vi "AB_UserComponentsPath.vi"(8 "error in (no error)":errorcluster) -> (0 "error out":errorcluster, 3 "path to User Components":path)   [LabVIEW 2020]
uses:
  <vilib>/registry/registry.llb/Registry View.ctl
  <vilib>/registry/registry.llb/Registry SAM.ctl
  <vilib>/registry/registry.llb/Registry RtKey.ctl
  <vilib>/registry/registry.llb/Read Registry Value Simple STR.vi
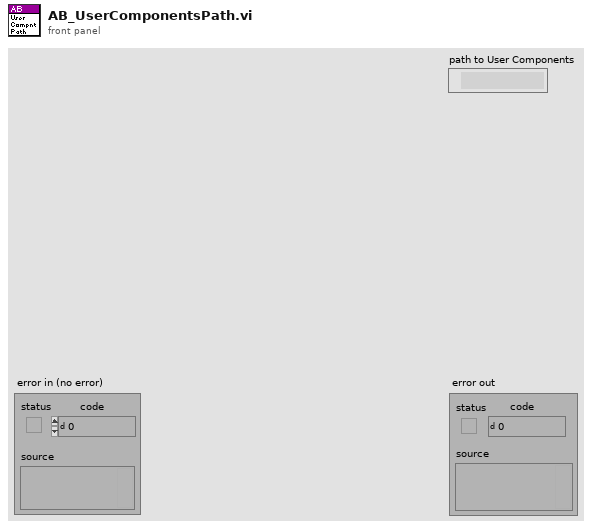
[diagram p1: front panel]
types:
  T1 = typedef "Registry RtKey.ctl" = enum32{"HKEY_CLASSES_ROOT", "HKEY_CURRENT_USER", "HKEY_LOCAL_MACHINE", "HKEY_USERS", "HKEY_PERFORMANCE_DATA", "HKEY_CURRENT_CONFIG", "HKEY_DYN_DATA"}
  T2 = typedef "Registry SAM.ctl" = enum32{"KEY_QUERY_VALUE", "KEY_SET_VALUE", "KEY_CREATE_SUB_KEY", "KEY_ENUMERATE_SUB_KEYS", "KEY_NOTIFY", "KEY_CREATE_LINK", "KEY_READ", "KEY_WRITE", "KEY_ALL_ACCESS", "KEY_READ | KEY_WRITE"}
  T3 = typedef "Registry View.ctl" = u16
  T4 = typedef "Registry refnum.ctl" = refnum<k1>
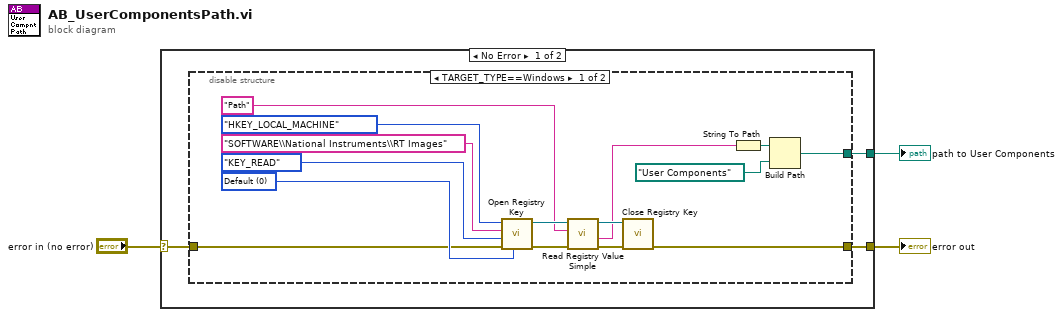
[diagram p0: block diagram]
diagram:
  n1 = case shown="No Error" "error in (no error)" {
    selector: "error in (no error)" -> [w5 w23]
    tunnel: [w6 w23] -> w3
    tunnel: [w4 _] -> w1
    frame No Error {
      n2 = disable-structure shown="TARGET_TYPE==Windows" {
        disable-tunnel: [w9 w22] -> w6
        disable-tunnel: w5 -> [w8 w22]
        disable-tunnel: [w7 _] -> w4
        frame condition #0 (active) {
          w16 = T3 0 items=["Default"=0, "KEY_WOW64_64KEY"=8, "KEY_WOW64_32KEY"=9] ("registry view")
          n3 = call <vilib>:"Open Registry Key.vi"("registry view"=w16, "error in (no error)"=w8, "security access mask (KEY_READ | KEY_WRITE)"=Registry_SAM."KEY_READ", "subkey"="SOFTWARE\\National Instruments\\RT Images", "root key (HKEY_LOCAL_MACHINE)"=Registry_RtKey."HKEY_LOCAL_MACHINE") -> ("error out"=w17:errorcluster, "refnum out"=w18:T4)  [unwired: 5 in]
          n4 = call-poly <vilib>:"Read Registry Value Simple.vi"("error in (no error)"=w17, "value"="Path", "refnum"=w18) -> ("error out"=w20:errorcluster, "String/Binary data"=w10:string, "refnum out"=w19:T4)  [unwired: 3 in, 1 out]
          n5 = call <vilib>:"Close Registry Key.vi"("error in (no error)"=w20, "refnum"=w19) -> ("error out"=w9:errorcluster)  [unwired: 5 in]
          n6 = String To Path(string=w10) -> (path=w11:path)
          n7 = Build Path(base path=w11, name or relative path=path "User Components") -> (appended path=w7:path)
        }
        frame condition #1 {
        }
      }
    }
    frame Error {
    }
  }
  "error out" <- w3
  "path to User Components" <- w1
